vi "Get IConfiguration.vi"(11 "DAQmx Base Configure Strategy in":refnum<class "DAQmx Base Configure Strategy.lvclass">) -> (2 "IConfiguration":refnum<class "IConfiguration.lvclass">, 3 "DAQmx Base Configure Strategy out":refnum<class "DAQmx Base Configure Strategy.lvclass">)   [LabVIEW 2024, in "DAQmx Base Configure Strategy.lvclass"]
uses:
  DAQmx Base Configure Strategy.lvclass
  Source/Interfaces/IConfiguration/IConfiguration.lvclass
  DAQmx Base Configure Strategy.lvclass/DAQmx Base Configure Strategy.ctl
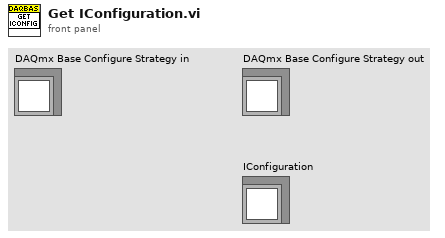
[diagram p1: front panel]
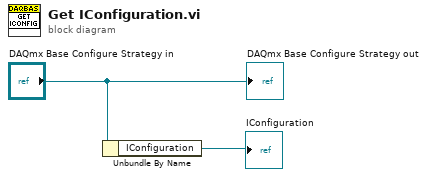
[diagram p0: block diagram]
diagram:
  n1 = Unbundle By Name("DAQmx Base Configure Strategy in") -> ("IConfiguration"=→"IConfiguration":refnum<class "IConfiguration.lvclass">)
  "DAQmx Base Configure Strategy out" <- "DAQmx Base Configure Strategy in"
